vi "Ist mit Soll vergleichen Regler.vi"(8 "error in (no error)":errorcluster caption="Fehler (Eingang, kein Fehler)", 10 "Index":u16, 11 "mini8 Steuerung PNS Eingang":refnum<class "mini8 Steuerung PNS.lvclass">) -> (0 "error out":errorcluster caption="Fehler (Ausgang)", 2 "Werte":cluster{u16[], u16[]}, 3 "mini8 Steuerung PNS Ausgang":refnum<class "mini8 Steuerung PNS.lvclass">)   [LabVIEW 2020, in "mini8 Steuerung PNS.lvclass"]
uses:
  mini8 Steuerung PNS.lvclass
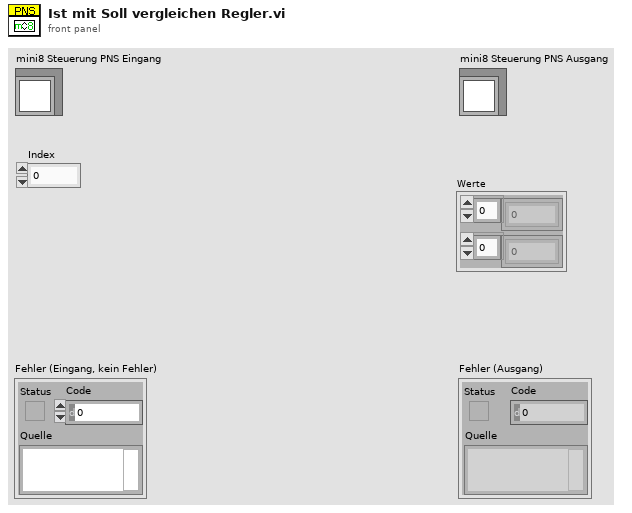
[diagram p1: front panel]
types:
  T1 = typedef "Steuerung PNS.lvclass/Anlegengrenzwerte PNS.ctl" = cluster{"Filter:":T2, "Ventilplatte:":T2, "Heizleitung 1:":T2, "Heizleitung 2:":T2, "Heizleitung 3:":T2, "Heizleitung 4:":T2, "Heizleitung 5:":T2, "Heizleitung 6:":T2}
  T2 = typedef "Steuerung PNS.lvclass/Anlagengrenzwerte Parameteranzeige.ctl" = cluster{"Sollwert":T3, "Warn-Min":T3, "Warn-Max":T3, "Abschalt-Min":T3, "Abschalt-Max":T3, "Regler":u16, "AnlagenParameter":string}
  T3 = typedef "Zahlen-Eingabefeld.ctl" = sgl
  T4 = typedef "Steuerung PNS.lvclass/Regler.ctl" = cluster{"Istwert":i16, "Sollwert":i16, "Alarm MIN":i16, "Alarm MAX":i16, "Regler sperren":i16, "Analog Ausgang":i16}[]
  T5 = cluster{"Istwert":i16, "Sollwert":i16, "Alarm MIN":i16, "Alarm MAX":i16, "Regler sperren":i16, "Analog Ausgang":i16}
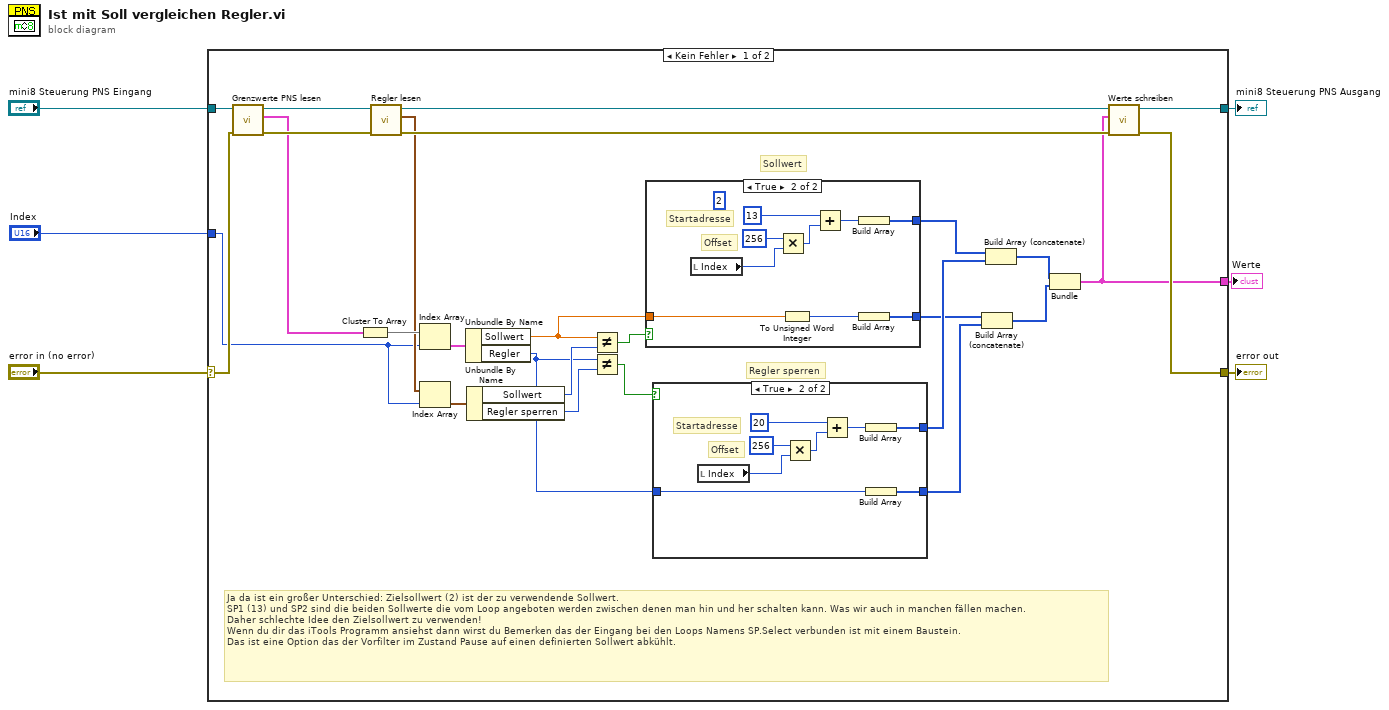
[diagram p0: block diagram]
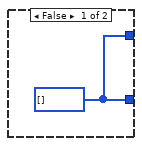
[diagram p2: hidden frame]
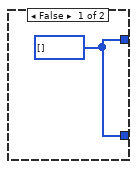
[diagram p3: hidden frame]
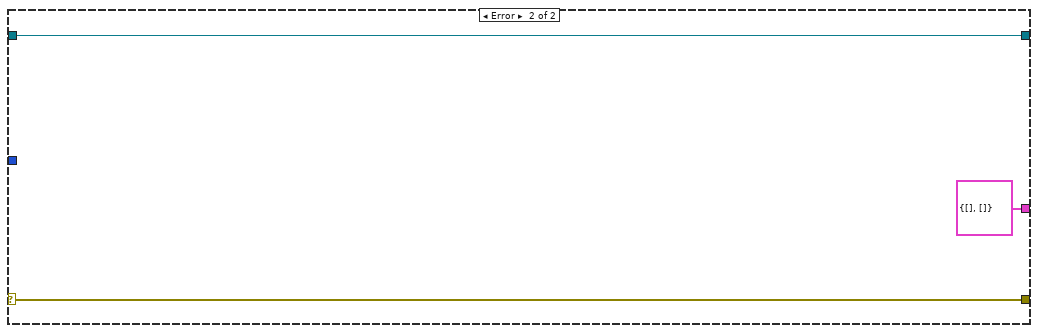
[diagram p4: hidden frame]
diagram:
  n1 = case shown="Kein Fehler" "error in (no error)" {
    selector: "error in (no error)" -> [w27 w55]
    tunnel: [w26 w55] -> w5
    tunnel: [w29 w54] -> w3
    tunnel: "mini8 Steuerung PNS Eingang" -> [w33 w54]
    tunnel: [w8 cluster{u16[], u16[]} {[], []}] -> w2
    tunnel: "Index" -> [w7 _]
    frame No Error {
      # "Ja da ist ein großer Unterschied: Zielsollwert (2) ist der zu verwendende Sollwert.\nSP1 (13) und SP2 sind die beiden Sollwerte die vom Loop angeboten werden zwischen denen man hin und her schalten kann. Was wir auch in manchen fällen machen. \nDaher schlechte Idee den Zielsollwert zu verwenden!\nWenn du dir das iTools Programm ansiehst dann wirst du Bemerken das der Eingang bei den Loops Namens SP.Select verbunden ist mit einem Baustein.\nDas ist eine Option das der Vorfilter im Zustand Pause auf einen definierten Sollwert abkühlt."
      # "Regler sperren"
      # "Sollwert"
      n2 = call-dynamic "Grenzwerte PNS lesen.vi"("error in (no error)"=w27, "Steuerung PNS (Eingang)"=w33) -> ("error out"=w30:errorcluster, "Grenzwerte PNS"=w12:T1, "Steuerung PNS (Ausgang)"=w32:refnum<class "mini8 Steuerung PNS.lvclass">)  [unwired: 7 in]
      n3 = Cluster To Array(cluster=w12) -> (array=w25:T2[])
      n4 = call-dynamic "Regler lesen.vi"("error in (no error)"=w30, "Steuerung PNS (Eingang)"=w32) -> ("error out"=w28:errorcluster, "Regler"=w11:T4, "Steuerung PNS (Ausgang)"=w31:refnum<class "mini8 Steuerung PNS.lvclass">)  [unwired: 7 in]
      n5 = Index Array(array=w25, index=w7) -> (element=w24:T2)
      n6 = Index Array(array=w11, index=w7) -> (element=w23:T5)
      n7 = Unbundle By Name(w24) -> ("Sollwert"=w19:T3, "Regler"=w18:u16)
      n8 = Unbundle By Name(w23) -> ("Sollwert"=w22:i16, "Regler sperren"=w21:i16)
      n9 = Not Equal?(x=w19, y=w22) -> (x != y?=w20:bool)
      n10 = Not Equal?(x=w18, y=w21) -> (x != y?=w17:bool)
      n11 = case shown="True" w20 {
        tunnel: w19 -> [_ w49]
        tunnel: [w43 w46] -> w16
        tunnel: [w43 w45] -> w14
        frame False {
          w43 = u16[] []
        }
        frame True {
          (unwired) u16 2
          # "Offset"
          # "Startadresse"
          n12 = local read "Index"() -> (w47:u16)
          n13 = Multiply(x=u16 256, y=w47) -> (x*y=w52:u16)
          n14 = To Unsigned Word Integer(number=w49) -> (unsigned 16bit integer=w48:u16)
          n15 = Add(x=u16 13, y=w52) -> (x+y=w50:u16)
          n16 = Build Array(w50) -> (w46:u16[])
          n17 = Build Array(w48) -> (w45:u16[])
        }
      }
      n18 = case shown="True" w17 {
        tunnel: w18 -> [_ w35]
        tunnel: [w34 w37] -> w15
        tunnel: [w34 w36] -> w13
        frame False {
          w34 = u16[] []
        }
        frame True {
          # "Offset"
          # "Startadresse"
          n19 = local read "Index"() -> (w38:u16)
          n20 = Multiply(x=u16 256, y=w38) -> (x*y=w42:u16)
          n21 = Add(x=u16 20, y=w42) -> (x+y=w39:u16)
          n22 = Build Array(w39) -> (w37:u16[])
          n23 = Build Array(w35) -> (w36:u16[])
        }
      }
      n24 = Build Array (concatenate)(w14, w13) -> (w10:u16[])
      n25 = Build Array (concatenate)(w16, w15) -> (w9:u16[])
      n26 = Bundle(w9, w10) -> (w8:cluster{u16[], u16[]})  [unwired: 1 in]
      n27 = call-dynamic "Werte schreiben.vi"("error in (no error)"=w28, "Werte"=w8, "Steuerung PNS (Eingang)"=w31) -> ("error out"=w26:errorcluster, "Steuerung PNS (Ausgang)"=w29:refnum<class "mini8 Steuerung PNS.lvclass">)  [unwired: 7 in]
    }
    frame Error {
    }
  }
  "error out" <- w5
  "mini8 Steuerung PNS Ausgang" <- w3
  "Werte" <- w2
